vi "SumMajoritySelectorIDInOut.vi"(5 "On Sum\nOff Majority":bool, 8 "error in":errorcluster, 10 "address":string="172.16.7.43", 11 "remote port or service name":u16=9764) -> (0 "error out":errorcluster={"status"=TRUE, "code"=63, "source"="TCP Open Connection in SumMajoritySelectorIDInOut.vi"})   [LabVIEW 2012]
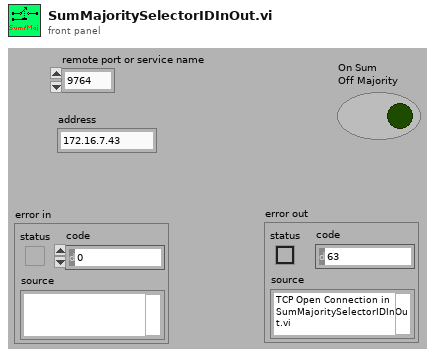
[diagram p1: front panel]
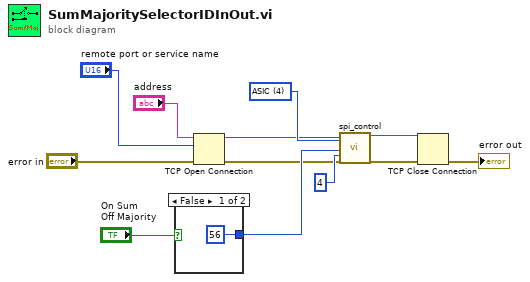
[diagram p0: block diagram]
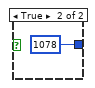
[diagram p2: hidden frame]
diagram:
  w12 = u16 4 items=["Attenuation", "Clipping", "Enable channel", "Delay line", "ASIC"] ("Device")
  n1 = case shown="False" "On Sum\nOff Majority" {
    tunnel: [56 ("Data") 1078 ("Data")] -> w10
    frame False {
    }
    frame True {
    }
  }
  n2 = TCP Open Connection(address="address", remote port or service name="remote port or service name", error in (no error)="error in") -> (connection ID=w4:refnum<k5>, error out=w6:errorcluster)  [unwired: 2 in]
  n3 = call "spi_control.vi"("connection ID"=w4, "Device"=w12, "Data"=w10, "Register or channel"=4, "error out 3"=w6) -> ("connection ID out"=w1:refnum<k5>, "error out 2"=w2:errorcluster)  [unwired: 7 in, 6 out]
  n4 = TCP Close Connection(connection ID=w1, error in (no error)=w2) -> (error out=→"error out":errorcluster)  [unwired: 1 in, 1 out]
